vi "RetVal.vi"() -> ()   [LabVIEW 2020]
panel:
  out "RetVal":bool
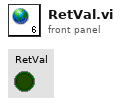
[diagram p1: front panel]
diagram:
